vi "输入员工ID.vi"(0 "Enable":bool=TRUE caption="启用", 5 "error in (no error)":errorcluster caption="错误输入（无错误）") -> (17 "输入员工ID":string, 18 "确定":bool, 19 "error out":errorcluster caption="错误输出")   [LabVIEW 2013]
doc: "显示标准对话框，提示用户输入用户名、密码等信息。\n--------------------\n\n该Express VI配置如下:\n\n显示给用户的信息:\n该输入为: \n文本输入框: 输入员工ID"
panel:
  in  "键盘":bool caption="OK1"
  in  "输入员工ID":string
  out "String":string caption="字符串"
  in  "Cancel":bool caption="取消"
  in  "OK2":bool
  in  "OK1":bool
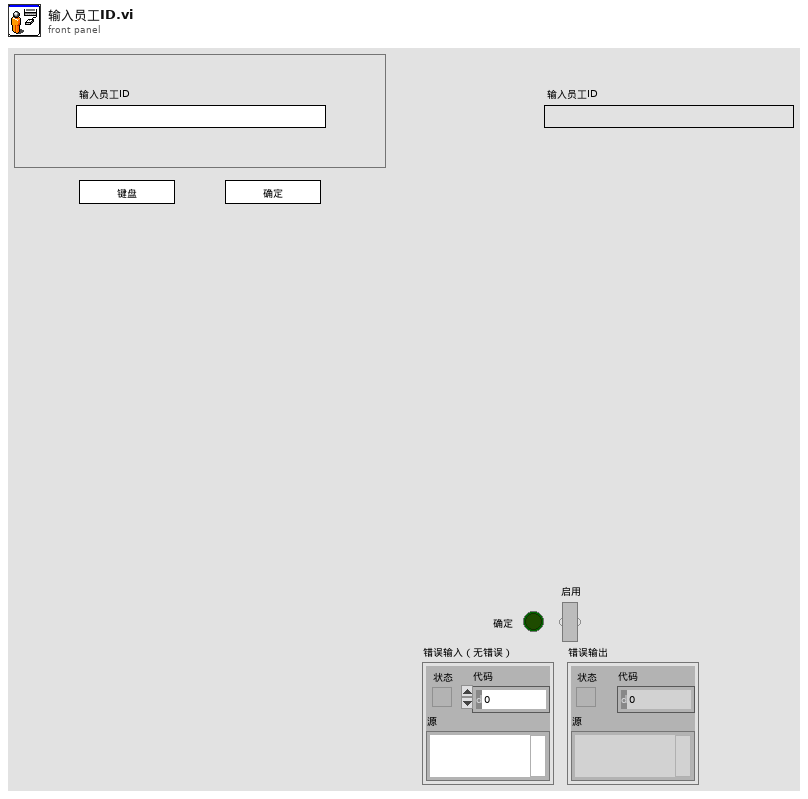
[diagram p1: front panel]
types:
  T1 = cluster{"Input Name":string, "Input Data Type":i32}[]
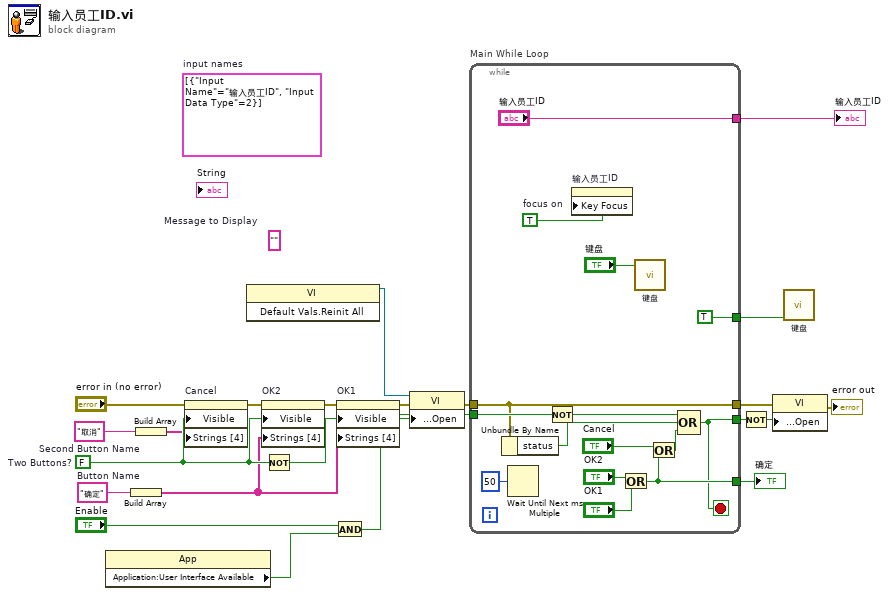
[diagram p0: block diagram]
diagram:
  (unwired) T1 [{"Input Name"="输入员工ID", "Input Data Type"=2}]  # input names
  w14 = "取消"  # Second Button Name
  w12 = "确定"  # Button Name
  (unwired) ""  # Message to Display
  w22 = FALSE  # Two Buttons?
  n1 = property class="App"() -> ("Application:User Interface Available"=w4:bool)  [unwired: 2 in, 2 out]
  n2 = Build Array(w12) -> (w13:string[])
  n3 = Build Array(w14) -> (w15:string[])
  n4 = property on="Cancel" class="Bool"(error in="error in (no error)", "Visible"=w22, "Strings [4]"=w15) -> (error out=w19:errorcluster)  [unwired: 1 in, 1 out]
  n5 = invoke class="VI" method="Default Vals.Reinit All"() -> (reference out=w3:refnum<vi>)  [unwired: 3 in, 2 out]
  n6 = property on="OK2" class="Bool"(error in=w19, "Visible"=w22, "Strings [4]"=w13) -> (error out=w18:errorcluster)  [unwired: 1 in, 1 out]
  n7 = Not(x=w22) -> (.not. x?=w20:bool)
  n8 = And(x="Enable", y=w4) -> (x .and. y?=w5:bool)
  n9 = property on="OK1" class="Bool"(error in=w18, "Visible"=w20, "Strings [4]"=w13) -> (error out=w11:errorcluster)  [unwired: 1 in, 1 out]
  n10 = property class="VI"(reference=w3, error in=w11, "Front Panel Window:Open"=w5) -> (error out=w10:errorcluster)  [unwired: 1 out]
  n11 = while "Main While Loop" {
    tunnel: [w34] -> w21
    tunnel: w5 -> [w32]
    tunnel: [w30] -> w16
    tunnel: w10 -> [w29]
    tunnel: [w29] -> w8
    tunnel: ["输入员工ID"] -> w2
    tunnel: [TRUE ("关闭")] -> w1
    stop <- w30 stop-if-true
    w23 = TRUE  # focus on
    n12 = Unbundle By Name(w29) -> ("status"=w27:bool)
    n13 = Wait Until Next ms Multiple(millisecond multiple=u32 50) -> ()  [unwired: 1 out]
    n14 = Not(x=w32) -> (.not. x?=w31:bool)
    n15 = property on="输入员工ID" class="Str"("Key Focus"=w23) -> ()  [unwired: 2 in, 2 out]
    n16 = Or(x="OK2", y="OK1") -> (x .or. y?=w34:bool)
    n17 = call "键盘.vi"("打开"="键盘") -> ()  [unwired: 3 in]
    n18 = Or(x="Cancel", y=w34) -> (x .or. y?=w28:bool)
    n19 = Compound Arithmetic op=OR(w31, w27, w28) -> (w30:bool)
  }
  "确定" <- w21
  "输入员工ID" <- w2
  n20 = Not(x=w16) -> (.not. x?=w17:bool)
  n21 = property class="VI"(error in=w8, "Front Panel Window:Open"=w17) -> (error out=→"error out":errorcluster)  [unwired: 1 in, 1 out]
  n22 = call "键盘.vi"("关闭"=w1) -> ()  [unwired: 3 in]
